vi "Update State String.vi"(8 "error in (no error)":errorcluster, 10 "State":string, 11 "Root Actor in":refnum<class "Root Actor.lvclass">) -> (0 "error out":errorcluster, 3 "Root Actor out":refnum<class "Root Actor.lvclass">)   [LabVIEW 2024, in "Root Actor.lvlib" / "Root Actor.lvclass"]
uses:
  Root Actor.lvclass
  Root Actor.lvclass/Root Actor.ctl
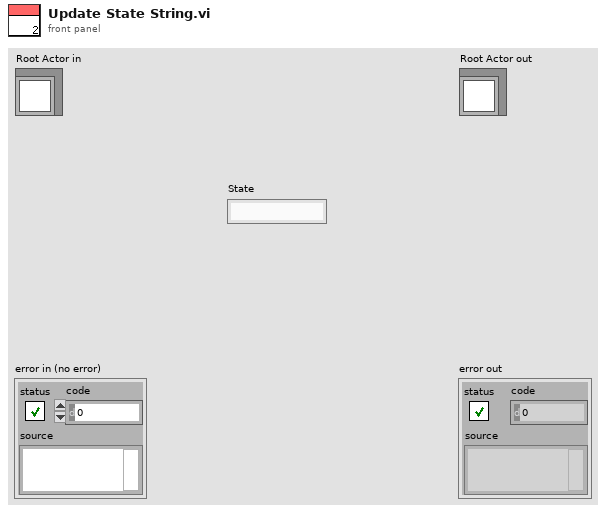
[diagram p1: front panel]
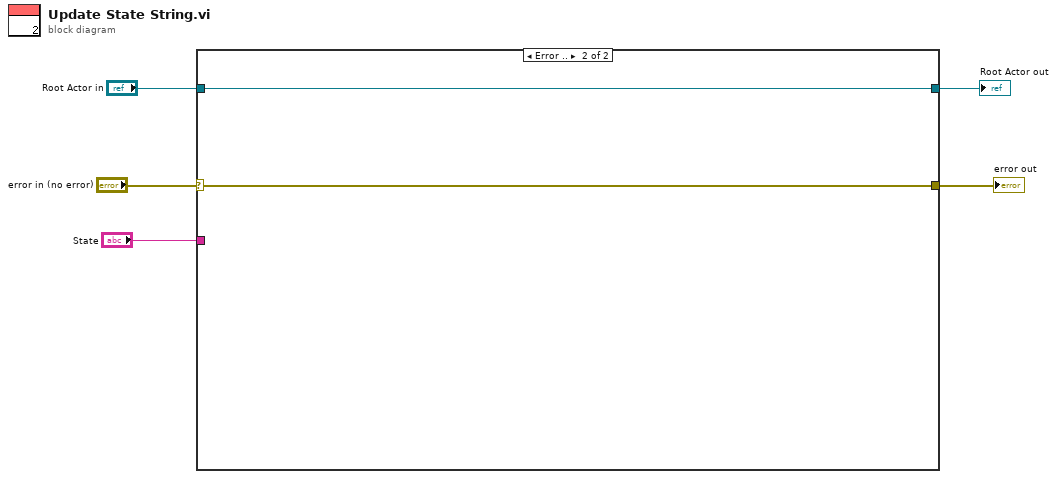
[diagram p0: block diagram]
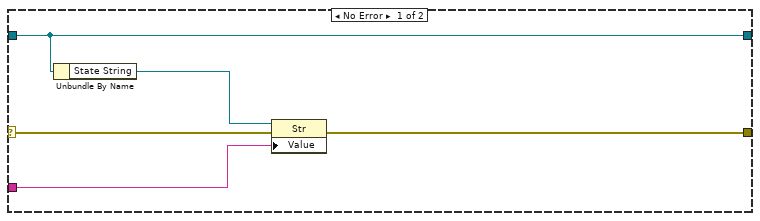
[diagram p2: hidden frame]
diagram:
  n1 = case shown="Error .." "error in (no error)" {
    selector: "error in (no error)" -> [w10 w11]
    tunnel: [w8 w11] -> w2
    tunnel: "Root Actor in" -> [w9 w12]
    tunnel: [w9 w12] -> w3
    tunnel: "State" -> [w6 _]
    frame No Error {
      n2 = Unbundle By Name(w9) -> ("State String"=w7:refnum<vi>)
      n3 = property class="Str"(reference=w7, error in=w10, "Value"=w6) -> (error out=w8:errorcluster)  [unwired: 1 out]
    }
    frame Error {
    }
  }
  "error out" <- w2
  "Root Actor out" <- w3
